vi "PaddleCor_V2.vi"() -> ()   [LabVIEW 2018]
uses:
  <vilib>/ptbypt/NI_PtbyPt.lvlib
panel:
  in  "Depth":dbl=1.5 step=0.1
  out "Waveform Chart 2":dbl(graph)
  out "True Interval (s)":dbl
  out "DeltaPaddle":dbl
  out "DeltaOut":dbl
  out "min out":dbl format="%0.2f"
  out "max out":dbl format="%0.2f"
  out "min paddle":dbl format="%0.2f"
  out "max paddle":dbl format="%0.2f"
  in  "Wave Period (sec)":dbl=0.5 min=0.5 step=0.1
  out "Driven Interval (s)":dbl=0.01 caption="Delay Time (s)" step=0.01
  in  "PID Gain":dbl(knob) scale=0.0..5.0
  in  "stop":bool
  in  "Sine Amplitude (cm)":dbl(knob) scale=0.0..10.0
  in  "Bias Voltage":dbl min=-0.2 max=0.0 step=0.01
  in  "Center Point (cm)":dbl=0.5 min=0.5 max=4.5 step=0.1
  out "Waveform Chart":dynamicdata(graph)
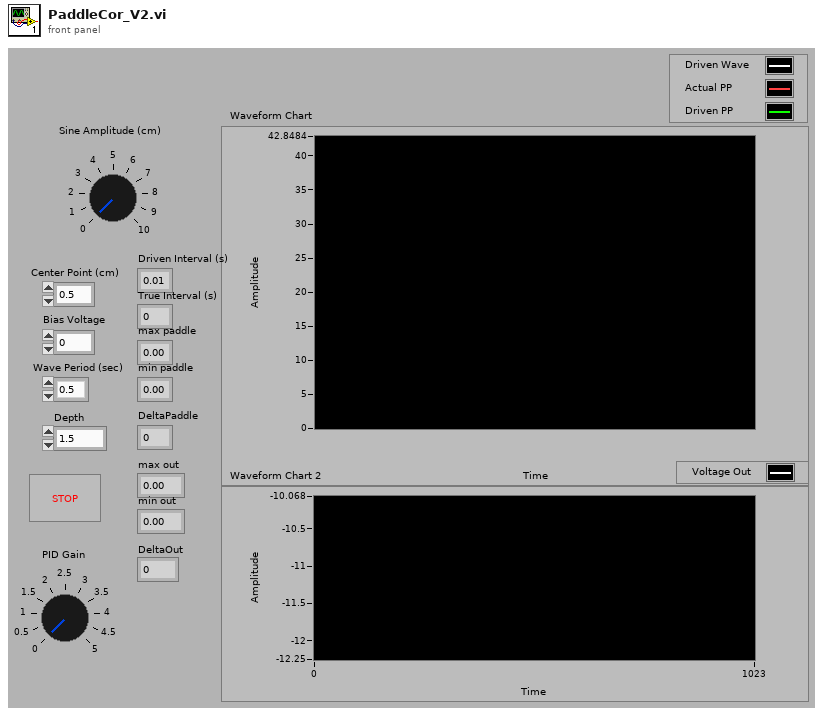
[diagram p1: front panel]
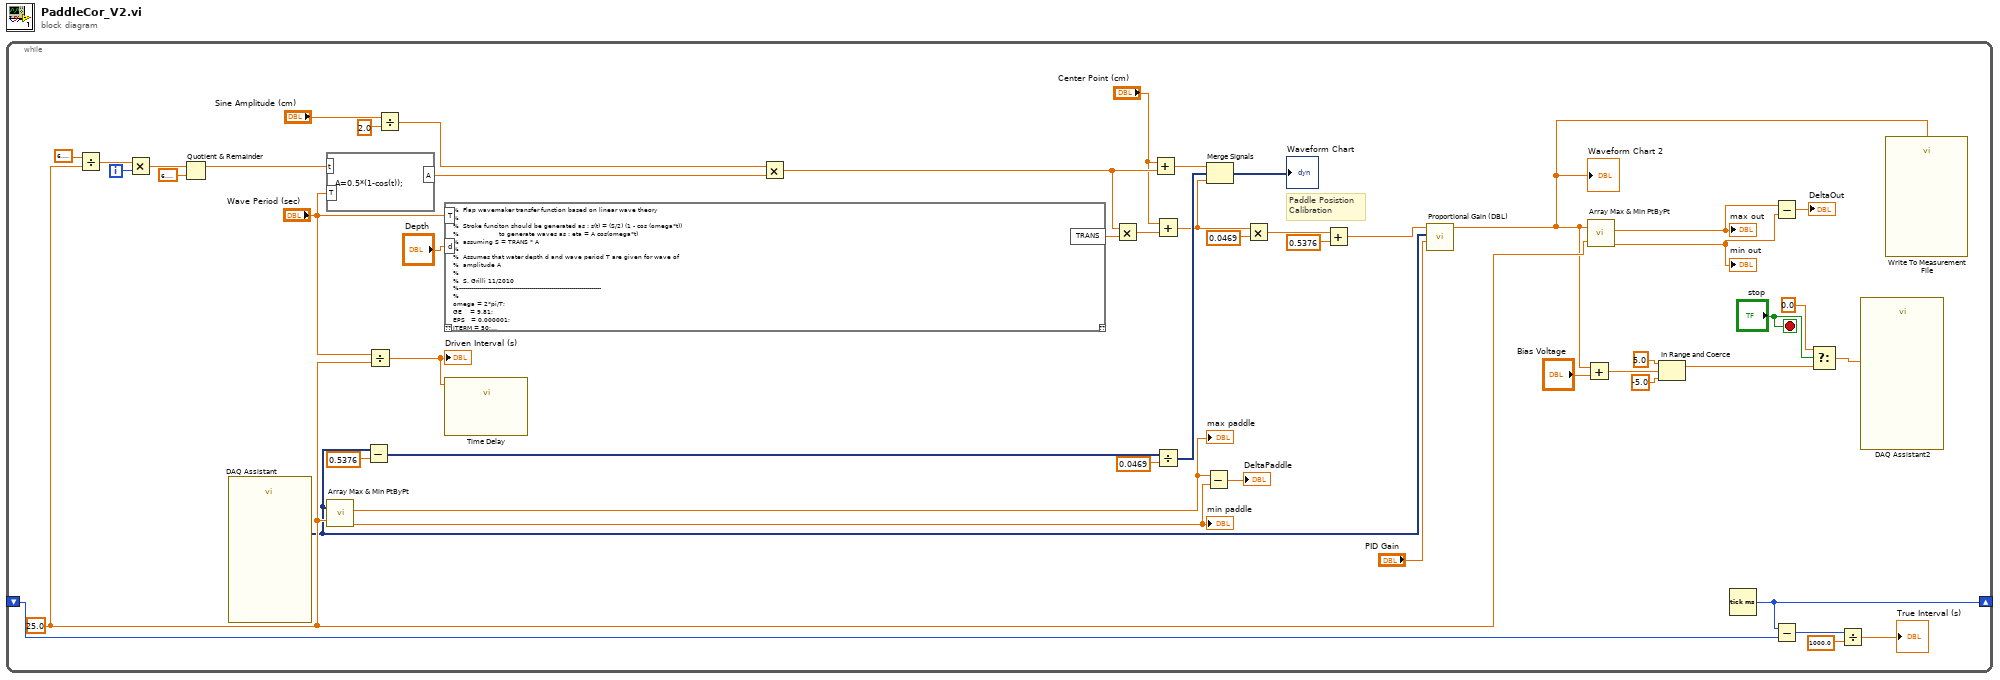
[diagram p0: block diagram]
diagram:
  n1 = while {
    shift-right: [w24] -> _
    shift-left: _ -> [w23]
    i -> [w49]
    stop <- "stop" stop-if-true
    w29 = 25.0 ("Resolution")
    # "Paddle Posistion\nCalibration"
    n2 = Divide(x=6.283185307179586, y=w29) -> (x/y=w50:dbl)
    n3 = Multiply(x=w50, y=w49) -> (x*y=w48:dbl)
    n4 = Quotient & Remainder(x=w48, y=6.283185307179586) -> (x-y*floor(x/y)=w3:dbl)  [unwired: 1 out]
    n5 = call "DAQ Assistant"() -> ("data"=w14:dynamicdata)  [unwired: 17 in, 2 out]
    n6 = formula code="A=0.5*(1-cos(t));"("t"=w3, "T"="Wave Period (sec)") -> ("A"=w2:dbl)
    n7 = call <vilib>:"Array Max & Min PtByPt.vi"("input data point"=w14, "sample length"=w29) -> ("max value"=w31:dbl, "min value"=w30:dbl)  [unwired: 1 in, 3 out]
    "max paddle" <- w31
    "min paddle" <- w30
    n8 = Subtract(x=w14, y=0.5376) -> (x-y=w13:dynamicdata)
    n9 = Divide(x="Wave Period (sec)", y=w29) -> (x/y=w28:dbl)
    "Driven Interval (s)" <- w28
    n10 = Divide(x="Sine Amplitude (cm)", y=2.0) -> (x/y=w21:dbl)
    n11 = script code="%  Flap wavemaker transfer function based on linear wave theory\n%\n%  Stroke funciton should be generated as : s(t) = (S/2) (1 - cos (omega*t))\n%                    to generate waves as : eta = A cos(omega*t)\n%  assuming S = TRANS * A\n%\n%  Assumes that water depth d and wave period T are given for wave of\n%  amplitude A\n%\n%  S. Grilli 11/2010\n%-----------------------------------------------------------------------\n%\nomega = 2*pi/T;  \nGE    = 9.81;\nEPS   = 0.000001;\nITERM = 50;   \n\n%.....Solves linear dispersion relationship\n\n      DE    = (omega.^2) .* d ./ GE;\n      ITER  = 0;  \n      ERR   = 1;\n%\n%.....Initial guess for nondimensional solution X\n%                                  \n      if (DE >= 1) \n         X0 = DE;\n      else\n         X0 = sqrt(DE);\n      end \n%\n%.....Solution using Newton-Raphson method\n%                    \n      while ((ERR > EPS) & (ITER <= ITERM))\n         F    = X0 - DE./tanh(X0);\n         DF   = 1 + DE./(sinh(X0).^2);\n         X1   = X0 - F./DF;\n         ERR  = abs((X1-X0)./X0);\n         X0   = X1;\n         ITER = ITER + 1;\n      end\n%\n      if (ITER > ITERM) \n         fprintf(1,'convergence failed\\r');                        \n      else\n         k = X1 / d;\n      end           \n      \ndt\t=\t1.925;  % depth to arm of hydraulic jack in meter (URI wavemaker)\nkd\t=\tk.*d;\nkd2\t=\t2*kd;\n\n% TRANS = So/H = So/(2A) as a function of (k,d) for linear flap hinged wavemaker (A=H/2)\n% and So is stroke amplitude\n\nTRANS =\t(kd2 + sinh(kd2))./(2.*sinh(kd).*(sinh(kd) + (1 - cosh(kd))./kd));\n\n% dt/d accounts for difference in water level d and hydraulic jack location \n% dt\n\nTRANS = TRANS.*dt./d;    %  This is now :  S/A"("T"="Wave Period (sec)", "d"="Depth") -> ("TRANS"=w10:dbl)  [unwired: 1 in, 1 out]
    n12 = call "Time Delay"("Delay Time (s)"=w28) -> ()  [unwired: 10 in, 1 out]
    n13 = Multiply(x=w21, y=w2) -> (x*y=w7:dbl)
    n14 = Multiply(x=w7, y=w10) -> (x*y=w8:dbl)
    n15 = Add(x="Center Point (cm)", y=w7) -> (x+y=w5:dbl)
    n16 = Add(x="Center Point (cm)", y=w8) -> (x+y=w9:dbl)
    n17 = Divide(x=w13, y=0.0469) -> (x/y=w12:dynamicdata)
    n18 = Subtract(x=w31, y=w30) -> (x-y=→"DeltaPaddle":dbl)
    n19 = Merge Signals "Merge Signals"(w5, w12, w9) -> (→"Waveform Chart":dynamicdata)
    n20 = Multiply(x=w9, y=0.0469) -> (x*y=w19:dbl)
    n21 = Add(x=w19, y=0.5376) -> (x+y=w18:dbl)
    n22 = call "Proportional Gain (DBL).vi"("Proportional Gain"="PID Gain", "Process Variable"=w14, "Set Point"=w18) -> ("Output Value"=w1:dbl)  [unwired: 8 in]
    "Waveform Chart 2" <- w1
    n23 = Add(x=w1, y="Bias Voltage") -> (x+y=w40:dbl)
    n24 = call <vilib>:"Array Max & Min PtByPt.vi"("input data point"=w1, "sample length"=w29) -> ("max value"=w35:dbl, "min value"=w34:dbl)  [unwired: 1 in, 3 out]
    "max out" <- w35
    "min out" <- w34
    n25 = In Range and Coerce(upper limit=5.0, x=w40, lower limit=-5.0) -> (coerced(x)=w39:dbl)  [unwired: 1 out]
    n26 = Tick Count (ms)() -> (millisecond timer value=w24:u32)
    n27 = Subtract(x=w35, y=w34) -> (x-y=→"DeltaOut":dbl)
    n28 = Subtract(x=w24, y=w23) -> (x-y=w26:u32)
    n29 = Select(t=0.0, s="stop", f=w39) -> (s? t:f=w36:dbl)
    n30 = Divide(x=w26, y=1000.0) -> (x/y=→"True Interval (s)":dbl)
    n31 = call "DAQ Assistant2"("data"=w36) -> ()  [unwired: 17 in, 2 out]
    n32 = call "Write To Measurement File"("Signals"=w1) -> ()  [unwired: 16 in, 3 out]
  }
